vi "counter 0-N.vi"(11 "reset":bool) -> (3 "iteration":fxp<+/-,32,32>)   [LabVIEW 2014]
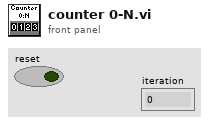
[diagram p1: front panel]
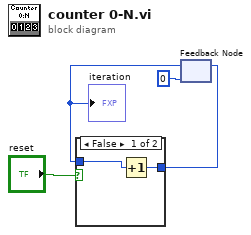
[diagram p0: block diagram]
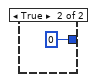
[diagram p2: hidden frame]
diagram:
  n1 = feedback #1(0) -> (w1:i32)
  "iteration" <- w1
  n2 = case shown="False" "reset" {
    tunnel: w1 -> [w6 _]
    tunnel: [w5 0] -> w3
    frame False {
      n3 = Increment(x=w6) -> (x+1=w5:i32)
    }
    frame True {
    }
  }
  n4 = feedback-in #1(w3) -> ()
